vi "Networktable comms.vi"   [LabVIEW 2014]
uses:
  AutonVars.vi
  Events.vi
  <vilib>/ptbypt/NI_PtbyPt.lvlib
panel:
  # "This is for all network table communications"
types:
  T1 = cluster{"OpJoyType":string, "DriveJoyType":string}
  T2 = cluster{"Translate":dbl, "Y-Axis (Backward Speed)":dbl, "Rotate":dbl, "Tank right side":dbl, "axis 5":dbl, "axis 6":dbl, "Use gyro":bool, "Exponential\ndrive":bool, "Ring light":bool, "PID rotation":bool, "PID Gain":dbl}
  T3 = cluster{"Reloading?":bool, "Throw":bool, "Ready?":bool, "Truss throw":bool, "Power is high?":bool, "Automatic relaod?":bool, "Manuall servo":bool}
  T4 = typedef "WPI_SolenoidValue.ctl" = enum16{"Off", "On", "Forward", "Reverse"}
  T5 = cluster{"Ultrasonic Distance (In)":dbl, "Gyro":dbl, "TopAquisition sensor":bool, "Encoder distance":dbl, "Encoder rate":dbl, "Encoder direction":bool, "winch engaged?":T4, "Motor Values":dbl[], "Latch encoder":u32, "BottomAquistion":bool, "BottomAquistion 2":bool, "Gyro Rate":dbl}
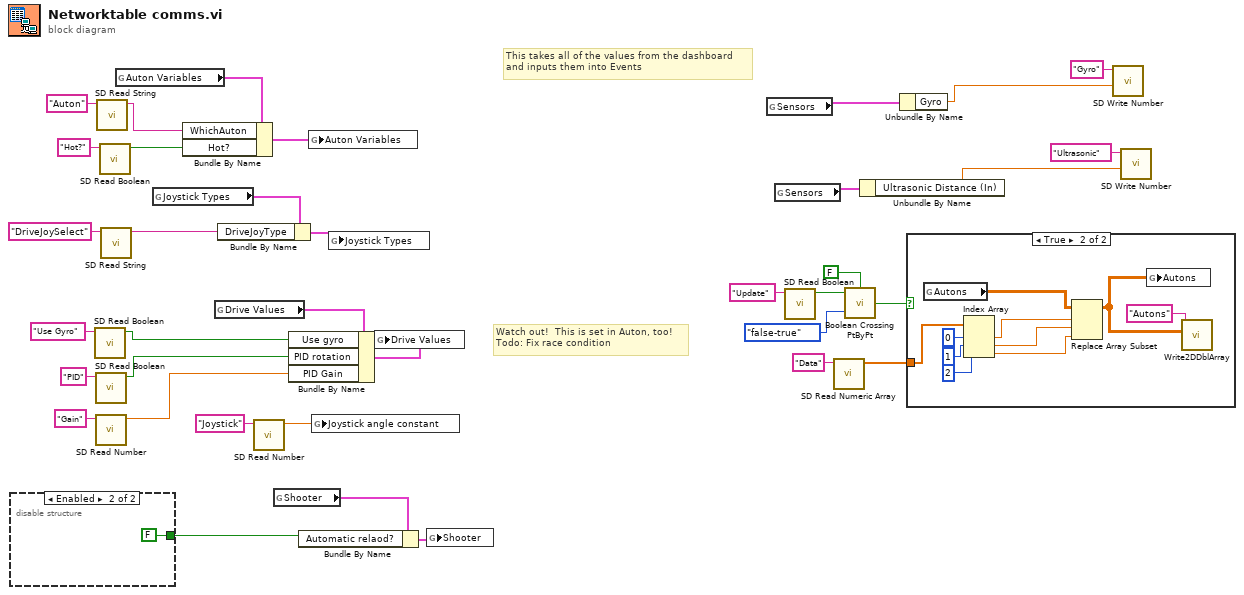
[diagram p0: block diagram]
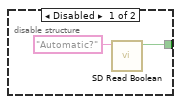
[diagram p2: hidden frame]
diagram:
  # "This takes all of the values from the dashboard\nand inputs them into Events"
  # "Watch out!  This is set in Auton, too!\nTodo: Fix race condition"
  n1 = disable-structure shown="Enabled" {
    disable-tunnel: [w38 FALSE] -> w24
    frame Disabled {
      n2 = call <vilib>:"SD Read Boolean.vi"("Name"="Automatic?") -> ("Boolean"=w38:bool)  [unwired: 8 in, 2 out]
    }
    frame Enabled {
    }
  }
  n3 = call <vilib>:"SD Read Boolean.vi"("Name"="Use Gyro") -> ("Boolean"=w30:bool)  [unwired: 8 in, 2 out]
  n4 = call <vilib>:"SD Read Boolean.vi"("Name"="PID") -> ("Boolean"=w5:bool)  [unwired: 8 in, 2 out]
  n5 = call <vilib>:"SD Read Number.vi"("Name"="Gain") -> ("Numeric"=w4:dbl)  [unwired: 8 in, 2 out]
  n6 = call <vilib>:"SD Read String.vi"("Name"="Auton") -> ("String"=w27:string)  [unwired: 8 in, 2 out]
  n7 = call <vilib>:"SD Read Boolean.vi"("Name"="Hot?") -> ("Boolean"=w34:bool)  [unwired: 8 in, 2 out]
  n8 = call <vilib>:"SD Read String.vi"("Name"="DriveJoySelect") -> ("String"=w9:string)  [unwired: 8 in, 2 out]
  n9 = global read "Events.vi" "Auton Variables"() -> (w35:cluster{"Hot?":bool, "WhichAuton":string})
  n10 = global read "Events.vi" "Joystick Types"() -> (w8:T1)
  n11 = Bundle By Name(cluster=w35, "WhichAuton"=w27, "Hot?"=w34) -> (w36:cluster{"Hot?":bool, "WhichAuton":string})
  n12 = global read "Events.vi" "Drive Values"() -> (w31:T2)
  n13 = Bundle By Name(cluster=w8, "DriveJoyType"=w9) -> (w7:T1)
  n14 = call <vilib>:"SD Read Number.vi"("Name"="Joystick") -> ("Numeric"=w2:dbl)  [unwired: 8 in, 2 out]
  n15 = global read "Events.vi" "Shooter"() -> (w25:T3)
  n16 = Bundle By Name(cluster=w31, "Use gyro"=w30, "PID rotation"=w5, "PID Gain"=w4) -> (w32:T2)
  n17 = Bundle By Name(cluster=w25, "Automatic relaod?"=w24) -> (w26:T3)
  n18 = global write "Events.vi" "Auton Variables"(w36) -> ()
  n19 = global write "Events.vi" "Joystick angle constant"(w2) -> ()
  n20 = global write "Events.vi" "Joystick Types"(w7) -> ()
  n21 = global write "Events.vi" "Drive Values"(w32) -> ()
  n22 = global write "Events.vi" "Shooter"(w26) -> ()
  n23 = global read "Events.vi" "Sensors"() -> (w22:T5)
  n24 = global read "Events.vi" "Sensors"() -> (w19:T5)
  n25 = call <vilib>:"SD Read Boolean.vi"("Name"="Update") -> ("Boolean"=w15:bool)  [unwired: 8 in, 2 out]
  n26 = call <vilib>:"SD Read Numeric Array.vi"("Name"="Data") -> ("Numeric Array"=w11:dbl[])  [unwired: 8 in, 2 out]
  n27 = call <vilib>:"Boolean Crossing PtByPt.vi"("initialize"=FALSE, "direction"=enum16{"either", "false-true", "true-false"}."false-true", "input"=w15) -> ("crossing"=w14:bool)
  n28 = Unbundle By Name(w19) -> ("Ultrasonic Distance (In)"=w18:dbl)
  n29 = Unbundle By Name(w22) -> ("Gyro"=w21:dbl)
  n30 = case shown="True" w14 {
    tunnel: w11 -> [_ w48]
    frame False {
    }
    frame True {
      n31 = global read "AutonVars.vi" "Autons"() -> (w49:dbl[][])
      n32 = Index Array(array=w48, index #1=0 ("index"), index #2=1 ("index"), index #3=2 ("index")) -> (element #1=w46:dbl, element #2=w44:dbl, element #3=w42:dbl)
      n33 = Replace Array Subset(array=w49, new element=w42, index (row)=w46, index (col)=w44) -> (w40:dbl[][])
      n34 = global write "AutonVars.vi" "Autons"(w40) -> ()
      n35 = call "Write2DDblArray.vi"("Write"=w40, "Name"="Autons") -> ()  [unwired: 8 in, 2 out]
    }
  }
  n36 = call <vilib>:"SD Write Number.vi"("Numeric"=w21, "Name"="Gyro") -> ()  [unwired: 8 in, 2 out]
  n37 = call <vilib>:"SD Write Number.vi"("Numeric"=w18, "Name"="Ultrasonic") -> ()  [unwired: 8 in, 2 out]
